vi "Read Tagged LLP Packet Cache.vi"(0 "state in":T1={"cache"=[0, 0, 0, 0, 0, 0, 0, 0, 0, 0, 0, 0, 0, 0, 0, 0], "cache size"=0.0, "state"=enum."wait for header", "end of packet"=FALSE}) -> (4 "state out":T1={"cache"=[0, 0, 0, 0, 0, 0, 0, 0, 0, 0, 0, 0, 0, 0, 0, 0], "cache size"=0.0, "state"=enum."wait for header", "end of packet"=FALSE}, 6 "serialized packet word":u8[](array[numeric]), 8 "valid bytes":fxp<+,4,4>, 10 "end of packet":bool)   [LabVIEW 2020, in "GettingStarted_Acq_Tap_148X_FPGA.lvlib"]
uses:
  <instrlib>/FlexRIO/CSI-2/v2/FPGA/Types/Serialize Tagged LLP Packet State Data.ctl
  <instrlib>/FlexRIO/CSI-2/v2/FPGA/Types/Serialize Tagged LLP Packet State.ctl
  GettingStarted_Acq_Tap_148X_FPGA.lvlib
  <instrlib>/FlexRIO/CSI-2/v2/FPGA/NI CSI-2 API FPGA v2.lvlib
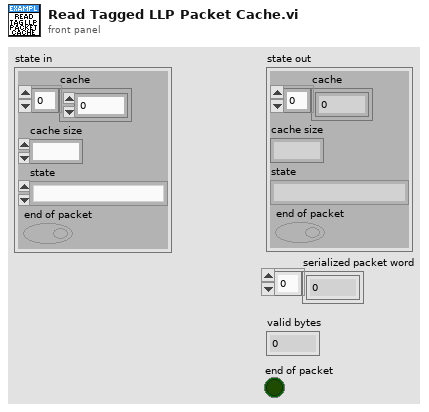
[diagram p1: front panel]
types:
  T1 = typedef "NI CSI-2 API FPGA v2.lvlib/Serialize Tagged LLP Packet State Data.ctl" = cluster{"cache":u8[], "cache size":fxp<+,5,5>, "state":T2, "end of packet":bool}
  T2 = typedef "NI CSI-2 API FPGA v2.lvlib/Serialize Tagged LLP Packet State.ctl" = enum8{"wait for header", "wait for end of packet"}
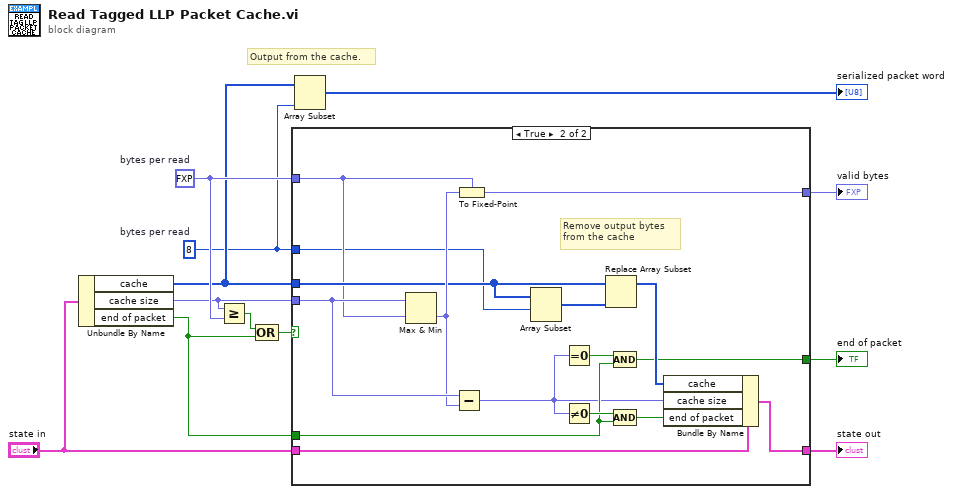
[diagram p0: block diagram]
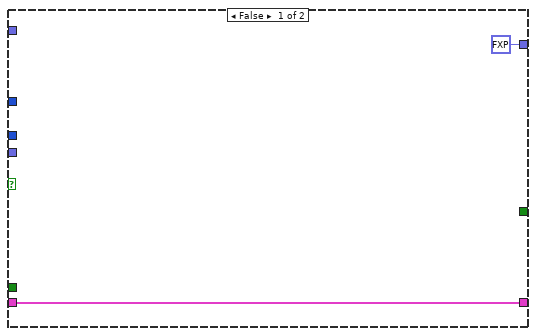
[diagram p2: hidden frame]
diagram:
  w3 = 8  # bytes per read
  w7 = fxp<+,4,4> 8.0  # bytes per read
  # "Output from the cache."
  n1 = Unbundle By Name("state in") -> ("cache"=w4:u8[], "cache size"=w6:fxp<+,5,5>, "end of packet"=w5:bool)
  n2 = Greater Or Equal?(x=w6, y=w7) -> (x >= y?=w8:bool)
  n3 = Compound Arithmetic op=OR(w8, w5) -> (w9:bool)
  n4 = case shown="True" w9 {
    tunnel: "state in" -> [w14 w30]
    tunnel: [fxp<+,3,3> 0.0 ("bytes per read") w29] -> w11
    tunnel: [w14 w28] -> w10
    tunnel: w6 -> [_ w27]
    tunnel: w4 -> [_ w23]
    tunnel: w7 -> [_ w22]
    tunnel: w3 -> [_ w21]
    tunnel: w5 -> [_ w18]
    tunnel: [_ w15] -> w1
    frame False {
    }
    frame True {
      # "Remove output bytes from the cache"
      n5 = Max & Min(x=w27, y=w22) -> (min(x,y)=w26:fxp<+,5,5>)  [unwired: 1 out]
      n6 = Subtract(x=w27, y=w26) -> (x-y=w17:fxp<+,5,5>)
      n7 = To Fixed-Point(fixed-point type=w22, number=w26) -> (fixed-point=w29:fxp<+,4,4>)
      n8 = Array Subset(array=w23, index=w21) -> (w24:u8[])  [unwired: 1 in]
      n9 = Equal To 0?(x=w17) -> (x = 0?=w16:bool)
      n10 = Not Equal To 0?(x=w17) -> (x != 0?=w19:bool)
      n11 = Replace Array Subset(array=w23, new element=w24) -> (w25:u8[])  [unwired: 1 in]
      n12 = Compound Arithmetic op=AND(w16, w18) -> (w15:bool)
      n13 = Compound Arithmetic op=AND(w19, w18) -> (w20:bool)
      n14 = Bundle By Name(cluster=w30, "cache"=w25, "cache size"=w17, "end of packet"=w20) -> (w28:T1)
    }
  }
  "valid bytes" <- w11
  "state out" <- w10
  "end of packet" <- w1
  n15 = Array Subset(array=w4, length=w3) -> (→"serialized packet word":u8[])  [unwired: 1 in]
